vi "no timeout error.vi"(1 "error in (no error)":errorcluster) -> (0 "error out":errorcluster)   [LabVIEW 2011]
doc: "When an error code is equal to 56 (time out error), the error cluster is initialized to 0 (no error)."
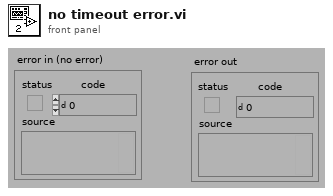
[diagram p1: front panel]
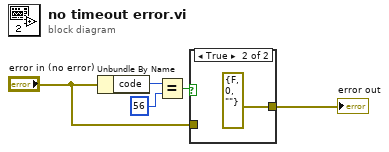
[diagram p0: block diagram]
diagram:
  n1 = Unbundle By Name("error in (no error)") -> ("code"=w5:i32)
  n2 = Equal?(x=w5, y=56) -> (x = y?=w3:bool)
  n3 = case shown="True" w3 {
    tunnel: "error in (no error)" -> [w6 _]
    tunnel: [w6 errorcluster {"status"=FALSE, "code"=0, "source"=""} ("error out")] -> w1
    frame False {
    }
    frame True {
    }
  }
  "error out" <- w1
